vi "质控内部交互全局.vi"() -> ()   [LabVIEW 2016, in "质控单元.lvlib"]
panel:
  out "database文件 path":path
  out "配置文件 path":path
  out "ping":bool
  in  "多个写入":T1={"starting address"=0, "values"=[], "Slave ID"=1}
  in  "仪器启动命令":T2={"仪器"=enum."氨氮", "starting address"=0, "value"=0}
  out "CODCr通讯状态":bool
  out "CODMn通讯状态":bool
  out "总氮通讯状态":bool
  out "总磷通讯状态":bool
  out "氨氮通讯状态":bool
  out "CODCr测量状态":u16[](array[numeric])
  out "CODMn测量状态":u16[](array[numeric])
  out "总氮测量状态":u16[](array[numeric])
  out "总磷测量状态":u16[](array[numeric])
  out "氨氮测量状态":u16[](array[numeric])
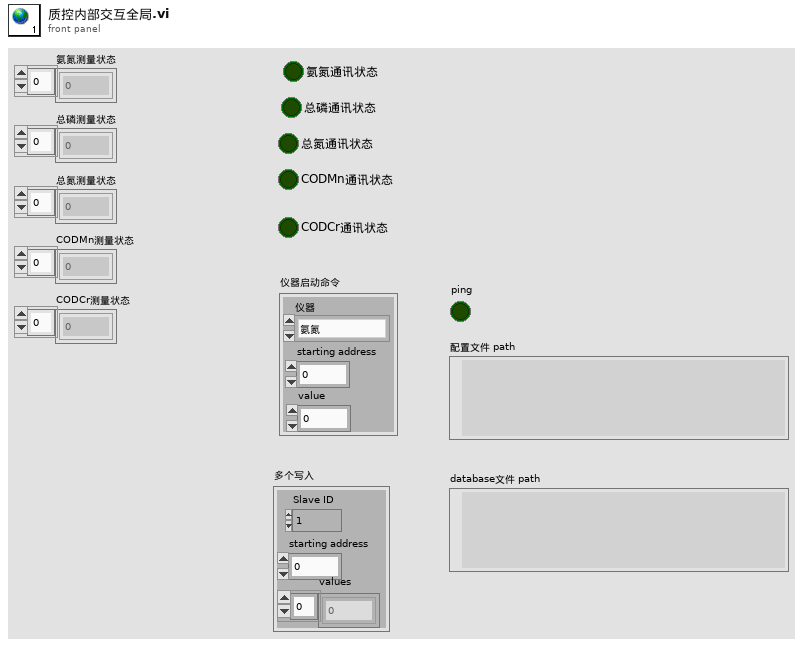
[diagram p1: front panel]
types:
  T1 = cluster{"starting address":u16, "values":u16[], "Slave ID":u8}
  T2 = cluster{"仪器":enum16{"", "氨氮", "总磷", "总氮", "CODMn", "CODCr"}, "starting address":u16, "value":u16}
diagram:
